vi "Logging Message Loop.vi"(8 "error in (no error)":errorcluster, 10 "Data Queue":refnum<queue>, 11 "Message Queues":T1) -> (0 "error out":errorcluster)   [LabVIEW 2022 SP3, in "Logging.lvlib"]
doc: "The message loop subVI to handle messages pertaining to logging data."
uses:
  Logging.lvlib
  support/Message Queue/All Message Queues.ctl
  support/Message Queue/Message Cluster.ctl
  Logging Configuration.ctl
  Logging State.ctl
  support/Message Queue/Enqueue Message (Single).vi
  <vilib>/Utility/error.llb/Error Cluster From Error Code.vi
  <vilib>/ErrorRing/Error Ring.xnode
  support/Message Queue/Message Queue.lvlib
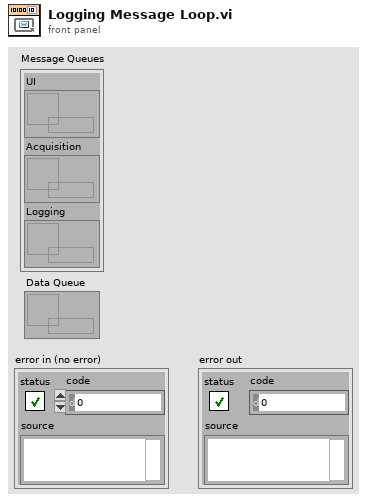
[diagram p1: front panel]
types:
  T1 = typedef "Message Queue.lvlib/All Message Queues.ctl" = cluster{"UI":refnum<queue>, "Acquisition":refnum<queue>, "Logging":refnum<queue>}
  T2 = typedef "Logging.lvlib/Logging Configuration.ctl" = cluster{"Log File Base Path":path, "*IDN?":string, "File Path Ref":refnum<file>, "Log Interval (s)":dbl, "Enable TimeStamp":bool, "Append File":bool}
  T3 = typedef "Logging.lvlib/Logging State.ctl" = enum16{"Idle", "Logging"}
  T4 = enum16{"open", "replace", "create", "open or create", "replace or create", "replace or create with confirmation"}
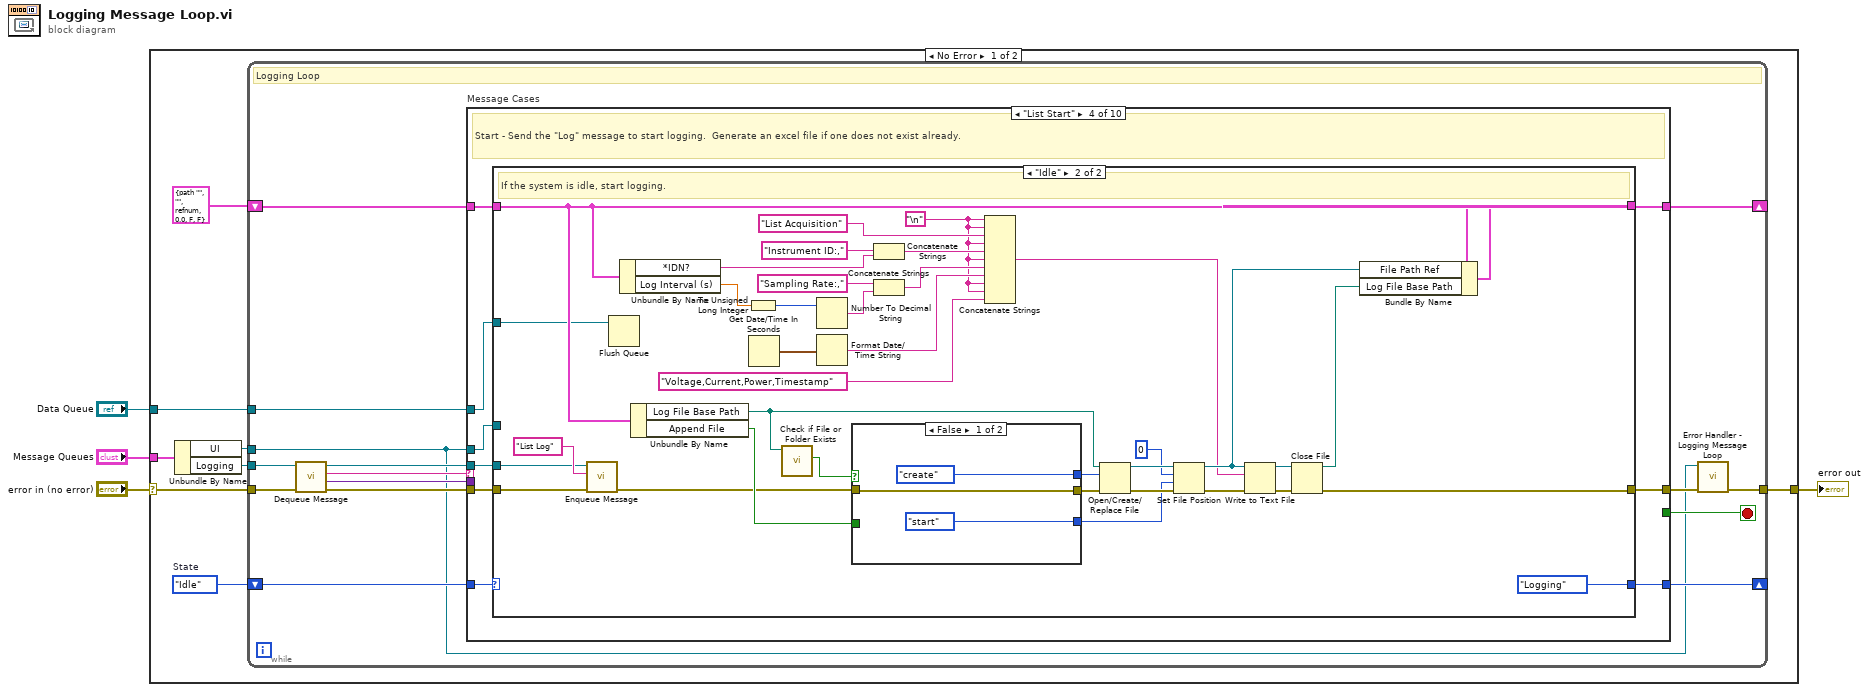
[diagram p0: block diagram]
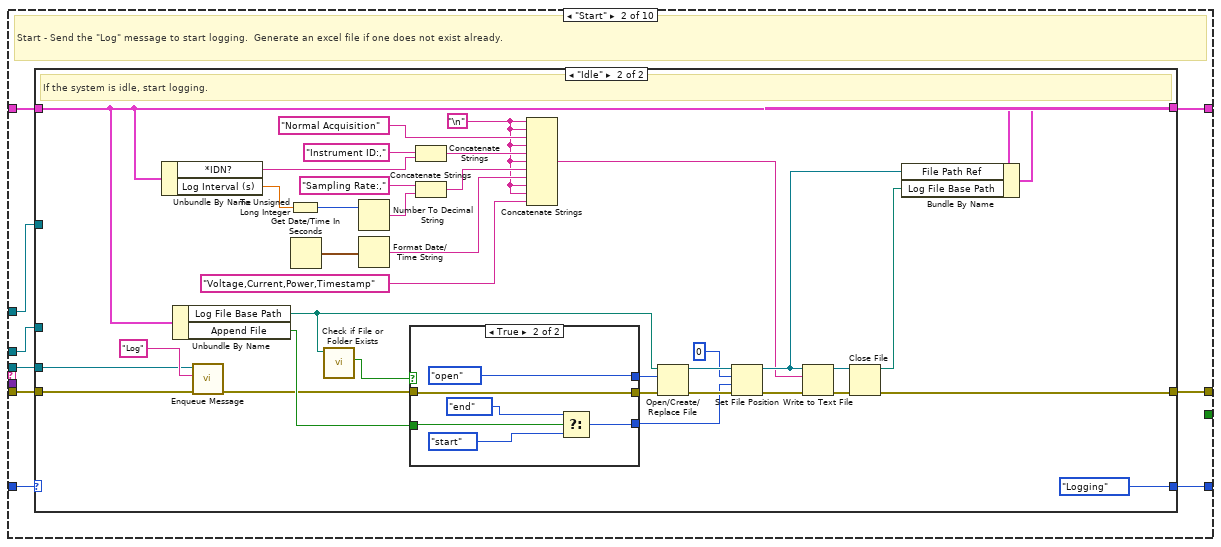
[diagram p3: hidden frame]
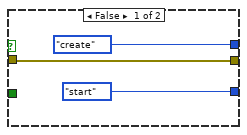
[diagram p5: hidden frame]
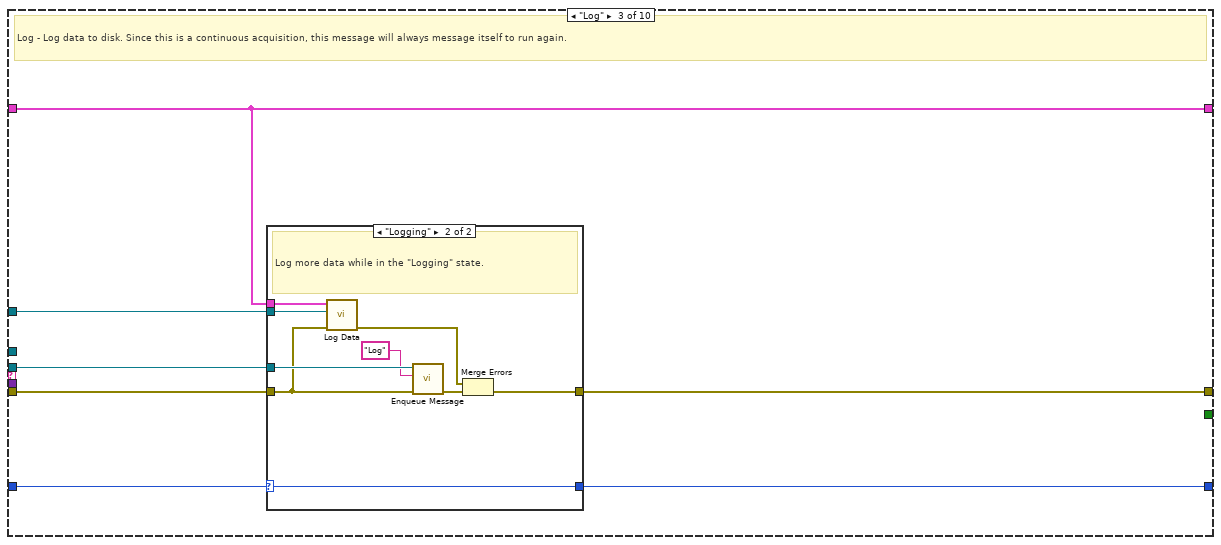
[diagram p6: hidden frame]
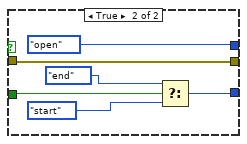
[diagram p9: hidden frame]
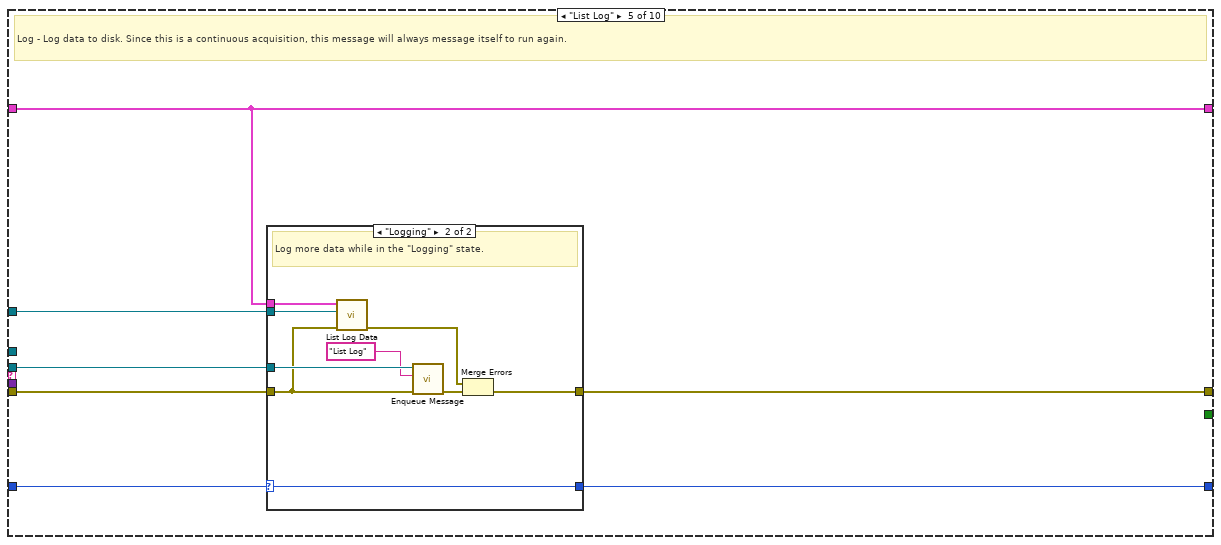
[diagram p10: hidden frame]
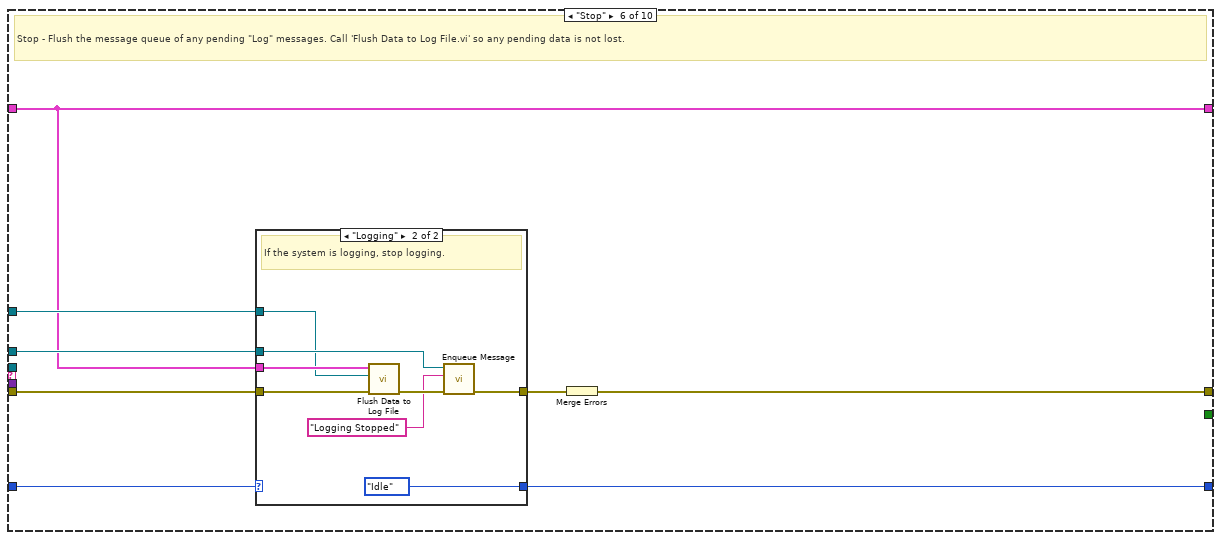
[diagram p12: hidden frame]
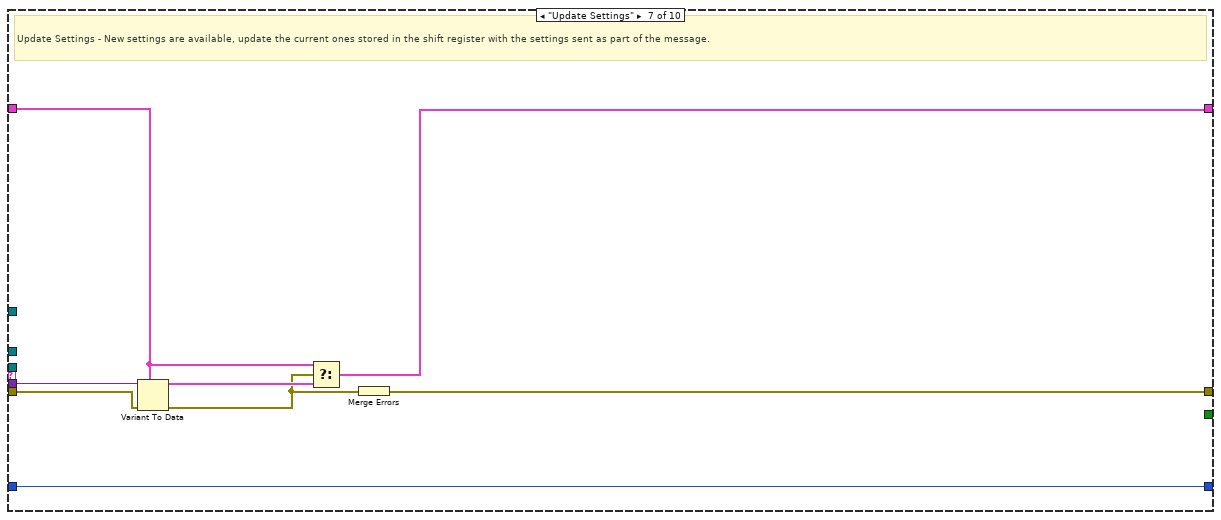
[diagram p14: hidden frame]
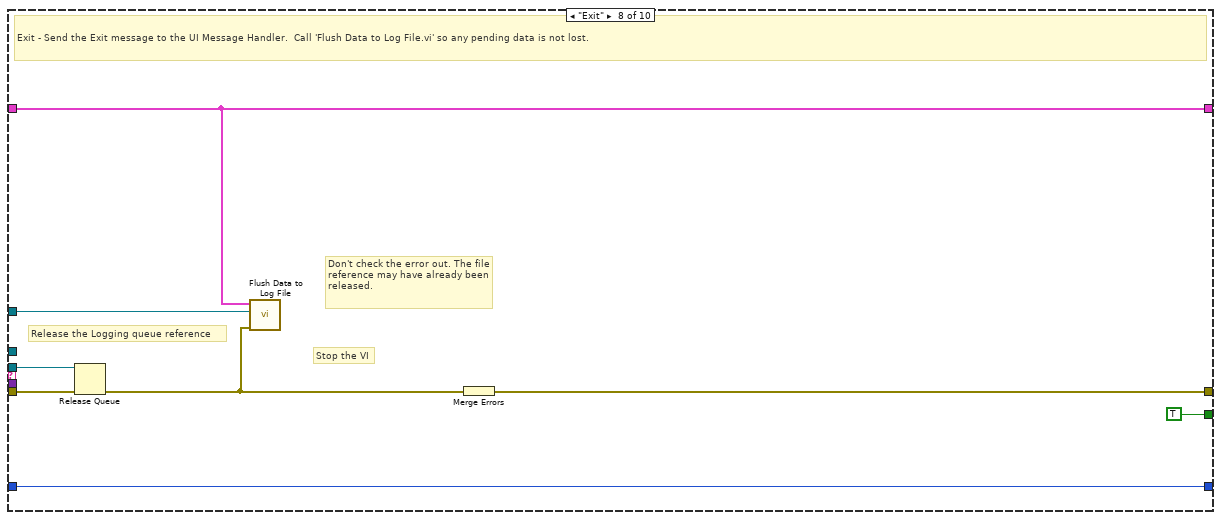
[diagram p15: hidden frame]
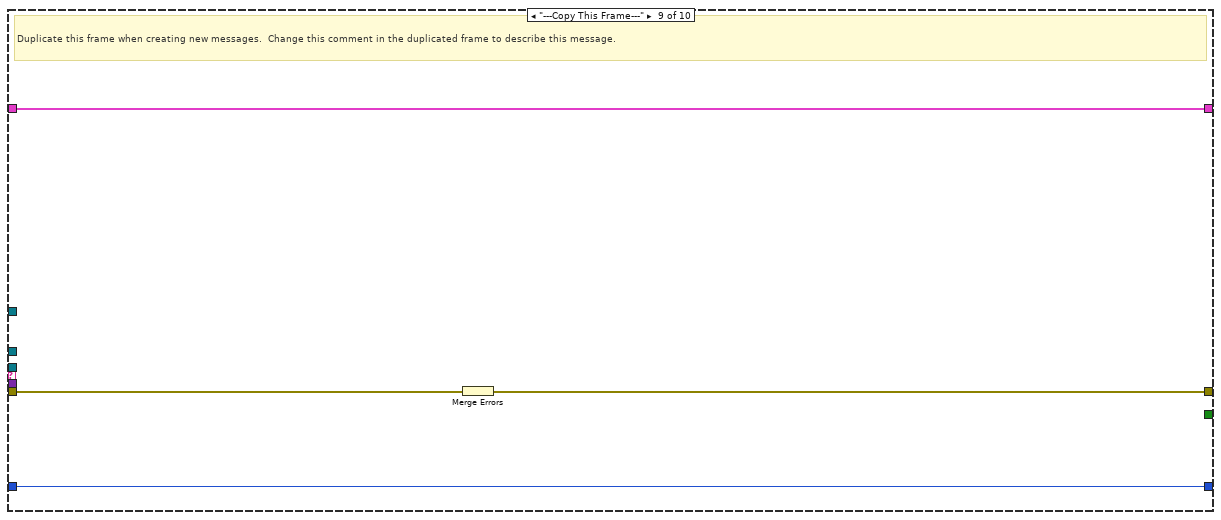
[diagram p16: hidden frame]
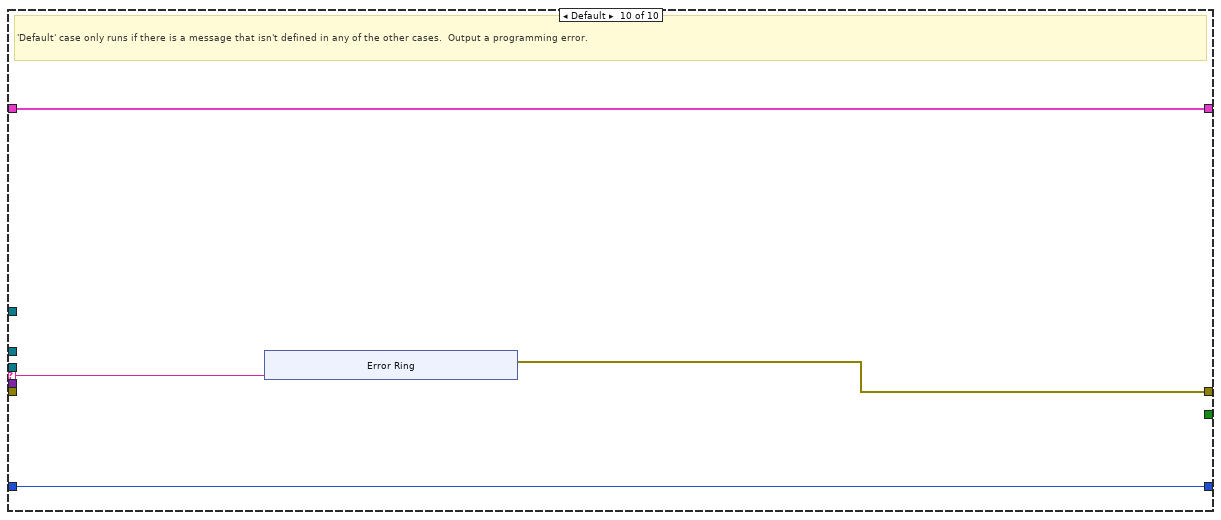
[diagram p17: hidden frame]
diagram:
  n1 = case shown="No Error" "error in (no error)" {
    selector: "error in (no error)" -> [w8 w231]
    tunnel: "Message Queues" -> [w12 _]
    tunnel: [w10 w231] -> w3
    tunnel: "Data Queue" -> [w5 _]
    frame No Error {
      w6 = Logging_State."Idle"  # State
      n2 = Unbundle By Name(w12) -> ("UI"=w7:refnum<queue>, "Logging"=w11:refnum<queue>)
      n3 = while {
        tunnel: w11 -> [w19]
        shift-right: [w26] -> _
        shift-left: T2 {"Log File Base Path"=path "", "*IDN?"="", "File Path Ref"=refnum, "Log Interval (s)"=0.0, "Enable TimeStamp"=FALSE, "Append File"=FALSE} ("Logging Configuration") -> [w27]
        tunnel: w7 -> [w14]
        shift-right: [w17] -> _
        shift-left: w6 -> [w18]
        tunnel: w8 -> [w24]
        tunnel: [w16] -> w10
        tunnel: w5 -> [w13]
        stop <- w25 stop-if-true
        # "Logging Loop"
        n4 = call "Dequeue Message.vi"("error in (no error)"=w24, "Message Queue"=w19) -> ("error out"=w23:errorcluster, "Message Data"=w21:variant, "Message"=w22:string, "dup Message Queue"=w20:refnum<queue>)  [unwired: 6 in]
        n5 = case "Message Cases" shown="\"List Start\"" w22 {
          selector: w22 -> [_ _ _ _ _ _ _ _ _ w220]
          tunnel: w20 -> [_ w38 w93 w113 w169 _ _ w212 _ _]
          tunnel: w23 -> [w29 w37 w91 w112 w168 w186 w202 w213 w219 _]
          tunnel: [w29 w39 w94 w114 w170 w189 w207 w214 w217 w221] -> w15
          tunnel: w27 -> [w30 w36 w90 w111 w167 w182 w205 w210 w218 w223]
          tunnel: [w30 w35 w90 w110 w167 w182 w203 w210 w218 w223] -> w26
          tunnel: [_ _ _ _ _ _ _ TRUE _ _] -> w25
          tunnel: w21 -> [_ _ _ _ _ _ w206 _ _ _]
          tunnel: w14 -> [_ w32 _ w107 _ w183 _ _ _ _]
          tunnel: w13 -> [_ w31 w92 w106 w164 w187 _ w209 _ _]
          tunnel: w18 -> [w28 w34 w89 w109 w166 w185 w201 w208 w216 w222]
          tunnel: [w28 w33 w88 w108 w165 w184 w201 w208 w216 w222] -> w17
          frame "Initialize" {
            # "Initialize - gets called when first launched. Currently a no-op."
          }
          frame "Start" {
            # "Start - Send the \"Log\" message to start logging.  Generate an excel file if one does not exist already."
            n6 = case shown="\"Idle\"" w34 {
              selector: w34 -> [w41 _]
              tunnel: [w40 w74] -> w39
              tunnel: w38 -> [_ w76]
              tunnel: w37 -> [w40 w77]
              tunnel: w36 -> [w42 w65]
              tunnel: [w42 w64] -> w35
              tunnel: [w41 Logging_State."Logging" ("State")] -> w33
              tunnel: w32 -> [_ _]
              tunnel: w31 -> [_ _]
              frame "Logging" {
                # "The system is already logging. Ignore the \"Start\" message."
              }
              frame "Idle" {
                w43 = "\n"
                # "If the system is idle, start logging."
                n7 = Unbundle By Name(w65) -> ("*IDN?"=w52:string, "Log Interval (s)"=w55:dbl)
                n8 = Unbundle By Name(w65) -> ("Log File Base Path"=w56:path, "Append File"=w62:bool)
                n9 = call-poly "Enqueue Message.vi"("error in (no error)"=w77, "Message"="Log", "Message Queue"=w76) -> ("error out"=w59:errorcluster)  [unwired: 7 in, 1 out]
                n10 = To Unsigned Long Integer(number=w55) -> (unsigned 32bit integer=w54:u32)
                n11 = Get Date/Time In Seconds() -> (seconds since 1Jan1904=w46:timestamp)
                n12 = call <vilib>:"Check if File or Folder Exists.vi"("path"=w56) -> ("file or folder exists?"=w60:bool)  [unwired: 8 in, 2 out]
                n13 = Number To Decimal String(number=w54) -> (decimal integer string=w49:string)  [unwired: 1 in]
                n14 = Format Date/Time String(seconds (now)=w46) -> (date/time string=w45:string)  [unwired: 2 in]
                n15 = case shown="True" w60 {
                  tunnel: [T4."create" ("operation (0:open)") T4."open" ("operation (0:open)")] -> w66
                  tunnel: w62 -> [_ w84]
                  tunnel: w59 -> [w80 w83]
                  tunnel: [w80 w83] -> w58
                  tunnel: [enum16{"start", "end", "current"}."start" ("from (0:start)") w82] -> w57
                  frame False {
                  }
                  frame True {
                    n16 = Select(t=enum16{"start", "end", "current"}."end" ("from (0:start)"), s=w84, f=enum16{"start", "end", "current"}."start" ("from (0:start)")) -> (s? t:f=w82:enum16{"start", "end", "current"})
                  }
                }
                n17 = Concatenate Strings("Instrument ID:,", w52) -> (w51:string)
                n18 = Concatenate Strings("Sampling Rate:,", w49) -> (w48:string)
                n19 = Concatenate Strings(w43, w43, "Normal Acquisition", w43, w51, w43, w48, w45, w43, w43, "Voltage,Current,Power,Timestamp" ("element")) -> (w61:string)
                n20 = Open/Create/Replace File(file path (use dialog)=w56, error in=w58, operation (0:open)=w66) -> (refnum out=w73:refnum<file>, error out=w72:errorcluster)  [unwired: 3 in, 1 out]
                n21 = Set File Position(offset (in bytes) (0)=i64 0, refnum=w73, from (0:start)=w57, error in=w72) -> (refnum out=w67:refnum<file>, error out=w71:errorcluster)
                n22 = Write to Text File(file (use dialog)=w67, text=w61, error in=w71) -> (refnum out=w69:refnum<file>, error out=w70:errorcluster)  [unwired: 1 in, 1 out]
                n23 = Close File(refnum=w69, error in=w70) -> (path=w75:path, error out=w74:errorcluster)
                n24 = Bundle By Name(cluster=w65, "File Path Ref"=w67, "Log File Base Path"=w75) -> (w64:T2)
              }
            }
          }
          frame "Log" {
            # "Log - Log data to disk. Since this is a continuous acquisition, this message will always message itself to run again."
            n25 = case shown="\"Logging\"" w89 {
              selector: w89 -> [w96 w98]
              tunnel: [w95 w105] -> w94
              tunnel: w93 -> [_ w103]
              tunnel: w92 -> [_ w102]
              tunnel: w91 -> [w95 w97]
              tunnel: w90 -> [_ w99]
              tunnel: [w96 w98] -> w88
              frame "Idle" {
                # "Ignore \"Log\" messages when the logging is idle."
              }
              frame "Logging" {
                # "Log more data while in the \"Logging\" state."
                n26 = call "Log Data.vi"("error in (no error)"=w97, "Data Queue"=w102, "Logging Configuration"=w99) -> ("error out"=w101:errorcluster)  [unwired: 8 in]
                n27 = call-poly "Enqueue Message.vi"("error in (no error)"=w97, "Message"="Log", "Message Queue"=w103) -> ("error out"=w104:errorcluster)  [unwired: 7 in, 1 out]
                n28 = Merge Errors(w101, w104) -> (w105:errorcluster)
              }
            }
          }
          frame "List Start" {
            # "Start - Send the \"Log\" message to start logging.  Generate an excel file if one does not exist already."
            n29 = case shown="\"Idle\"" w109 {
              selector: w109 -> [w116 _]
              tunnel: [w115 w150] -> w114
              tunnel: w113 -> [_ w152]
              tunnel: w112 -> [w115 w153]
              tunnel: w111 -> [w117 w141]
              tunnel: [w117 w140] -> w110
              tunnel: [w116 Logging_State."Logging" ("State")] -> w108
              tunnel: w107 -> [_ _]
              tunnel: w106 -> [_ w135]
              frame "Logging" {
                # "The system is already logging. Ignore the \"Start\" message."
              }
              frame "Idle" {
                w118 = "\n"
                # "If the system is idle, start logging."
                n30 = call-poly "Enqueue Message.vi"("error in (no error)"=w153, "Message"="List Log", "Message Queue"=w152) -> ("error out"=w134:errorcluster)  [unwired: 7 in, 1 out]
                n31 = Flush Queue(queue=w135) -> ()  [unwired: 1 in, 3 out]
                n32 = Unbundle By Name(w141) -> ("*IDN?"=w127:string, "Log Interval (s)"=w130:dbl)
                n33 = Unbundle By Name(w141) -> ("Log File Base Path"=w131:path, "Append File"=w138:bool)
                n34 = To Unsigned Long Integer(number=w130) -> (unsigned 32bit integer=w129:u32)
                n35 = Get Date/Time In Seconds() -> (seconds since 1Jan1904=w121:timestamp)
                n36 = call <vilib>:"Check if File or Folder Exists.vi"("path"=w131) -> ("file or folder exists?"=w136:bool)  [unwired: 8 in, 2 out]
                n37 = Number To Decimal String(number=w129) -> (decimal integer string=w124:string)  [unwired: 1 in]
                n38 = Format Date/Time String(seconds (now)=w121) -> (date/time string=w120:string)  [unwired: 2 in]
                n39 = case shown="False" w136 {
                  tunnel: [T4."create" ("operation (0:open)") T4."open" ("operation (0:open)")] -> w142
                  tunnel: w138 -> [_ w160]
                  tunnel: w134 -> [w156 w159]
                  tunnel: [w156 w159] -> w133
                  tunnel: [enum16{"start", "end", "current"}."start" ("from (0:start)") w158] -> w132
                  frame False {
                  }
                  frame True {
                    n40 = Select(t=enum16{"start", "end", "current"}."end" ("from (0:start)"), s=w160, f=enum16{"start", "end", "current"}."start" ("from (0:start)")) -> (s? t:f=w158:enum16{"start", "end", "current"})
                  }
                }
                n41 = Concatenate Strings("Instrument ID:,", w127) -> (w126:string)
                n42 = Concatenate Strings("Sampling Rate:,", w124) -> (w123:string)
                n43 = Concatenate Strings(w118, w118, "List Acquisition", w118, w126, w118, w123, w120, w118, w118, "Voltage,Current,Power,Timestamp" ("element")) -> (w137:string)
                n44 = Open/Create/Replace File(file path (use dialog)=w131, error in=w133, operation (0:open)=w142) -> (refnum out=w149:refnum<file>, error out=w148:errorcluster)  [unwired: 3 in, 1 out]
                n45 = Set File Position(offset (in bytes) (0)=i64 0, refnum=w149, from (0:start)=w132, error in=w148) -> (refnum out=w143:refnum<file>, error out=w147:errorcluster)
                n46 = Write to Text File(file (use dialog)=w143, text=w137, error in=w147) -> (refnum out=w145:refnum<file>, error out=w146:errorcluster)  [unwired: 1 in, 1 out]
                n47 = Close File(refnum=w145, error in=w146) -> (path=w151:path, error out=w150:errorcluster)
                n48 = Bundle By Name(cluster=w141, "File Path Ref"=w143, "Log File Base Path"=w151) -> (w140:T2)
              }
            }
          }
          frame "List Log" {
            # "Log - Log data to disk. Since this is a continuous acquisition, this message will always message itself to run again."
            n49 = case shown="\"Logging\"" w166 {
              selector: w166 -> [w172 w177]
              tunnel: [w171 w181] -> w170
              tunnel: w169 -> [_ w179]
              tunnel: w168 -> [w171 w176]
              tunnel: w167 -> [_ w174]
              tunnel: [w172 w177] -> w165
              tunnel: w164 -> [_ w173]
              frame "Idle" {
                # "Ignore \"Log\" messages when the logging is idle."
              }
              frame "Logging" {
                # "Log more data while in the \"Logging\" state."
                n50 = call "List Log Data.vi"("error in (no error)"=w176, "Data Queue"=w173, "Logging Configuration"=w174) -> ("error out"=w175:errorcluster)  [unwired: 8 in]
                n51 = call-poly "Enqueue Message.vi"("error in (no error)"=w176, "Message"="List Log", "Message Queue"=w179) -> ("error out"=w180:errorcluster)  [unwired: 7 in, 1 out]
                n52 = Merge Errors(w175, w180) -> (w181:errorcluster)
              }
            }
          }
          frame "Stop" {
            # "Stop - Flush the message queue of any pending \"Log\" messages. Call 'Flush Data to Log File.vi' so any pending data is not lost."
            n53 = case shown="\"Logging\"" w185 {
              selector: w185 -> [w190 _]
              tunnel: [w191 w195] -> w188
              tunnel: w187 -> [_ w192]
              tunnel: w182 -> [_ w198]
              tunnel: w186 -> [w191 w197]
              tunnel: [w190 Logging_State."Idle" ("State")] -> w184
              tunnel: w183 -> [_ w194]
              frame "Idle" {
                # "The system is already idle. Ignore the \"Stop\" message."
              }
              frame "Logging" {
                # "If the system is logging, stop logging."
                n54 = call "Flush Data to Log File.vi"("error in (no error)"=w197, "Data Queue"=w192, "Logging Configuration"=w198) -> ("error out"=w199:errorcluster)  [unwired: 8 in]
                n55 = call-poly "Enqueue Message.vi"("error in (no error)"=w199, "Message"="Logging Stopped", "Message Queue"=w194) -> ("error out"=w195:errorcluster)  [unwired: 7 in, 1 out]
              }
            }
            n56 = Merge Errors(w188) -> (w189:errorcluster)
          }
          frame "Update Settings" {
            # "Update Settings - New settings are available, update the current ones stored in the shift register with the settings sent as part of the message."
            n57 = Variant To Data(error in=w202, type=w205, Variant=w206) -> (data=w204:T2, error out=w200:errorcluster)
            n58 = Select(t=w205, s=w200, f=w204) -> (s? t:f=w203:T2)
            n59 = Merge Errors(w200) -> (w207:errorcluster)
          }
          frame "Exit" {
            # "Don't check the error out. The file reference may have already been released."
            # "Release the Logging queue reference"
            # "Stop the VI"
            # "Exit - Send the Exit message to the UI Message Handler.  Call 'Flush Data to Log File.vi' so any pending data is not lost."
            n60 = Release Queue(queue=w212, error in (no error)=w213) -> (error out=w211:errorcluster)  [unwired: 1 in, 2 out]
            n61 = call "Flush Data to Log File.vi"("error in (no error)"=w211, "Data Queue"=w209, "Logging Configuration"=w210) -> ()  [unwired: 8 in, 1 out]
            n62 = Merge Errors(w211) -> (w214:errorcluster)
          }
          frame "---Copy This Frame---" {
            # "Duplicate this frame when creating new messages.  Change this comment in the duplicated frame to describe this message."
            n63 = Merge Errors(w219) -> (w217:errorcluster)
          }
          frame Default {
            # "'Default' case only runs if there is a message that isn't defined in any of the other cases.  Output a programming error."
            n64 = xnode "Error Ring"("parameter 0"=w220) -> ("error out"=w221:errorcluster)
          }
        }
        n65 = call "Error Handler - Logging Message Loop.vi"("error in (no error)"=w15, "Message Queue"=w14) -> ("dup error in"=w16:errorcluster)  [unwired: 8 in, 1 out]
      }
    }
    frame Error {
    }
  }
  "error out" <- w3
